vi "Command (read) - IV.vi"(7 "timeout ms (100)":i32=100, 8 "error in (no error)":errorcluster, 9 "Paremeter":string, 10 "IP":string, 11 "connection ID in":refnum<k16>) -> (0 "error out":errorcluster, 2 "Velocity":dbl, 3 "connection ID out":refnum<k16>)   [LabVIEW 2016, in "SMD-7615.lvlib" / "eSCL.lvlib"]
doc: "IV - Immediate Velocity\nRequests present velocity of the motor in rpm. There are two different velocities that can be read back: the\nmotor’s actual velocity and the motor’s target velocity.\nParameter : \n0 = actual velocity request (servo drives and stepper drives with encoder)\n1 = target velocity request"
uses:
  eSCL.lvlib
  DBL Command and Param.ctl
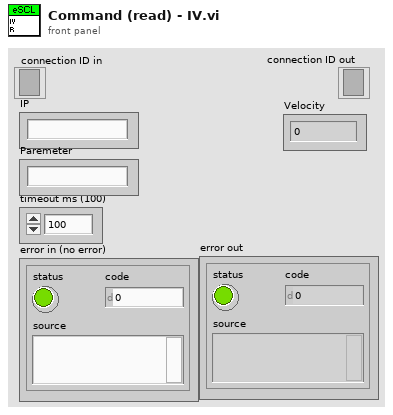
[diagram p1: front panel]
types:
  T1 = typedef "SMD-7615.lvlib/eSCL.lvlib/DBL Command and Param.ctl" = cluster{"Command":string, "DBL Parameler":dbl, "DBL Parameler Default":dbl, "DBL Parameler Coerece Upper":dbl, "DBL Parameler Coerece Lower":dbl}
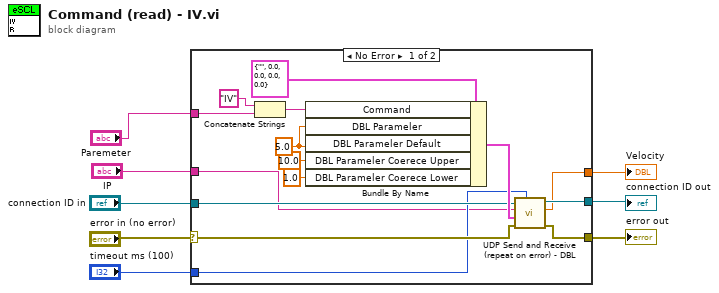
[diagram p0: block diagram]
diagram:
  n1 = case shown="No Error" "error in (no error)" {
    selector: "error in (no error)" -> [w19 w25]
    tunnel: [w18 w24] -> w7
    tunnel: [w17 w25] -> w5
    tunnel: [w16 _] -> w6
    tunnel: "connection ID in" -> [w12 w24]
    tunnel: "timeout ms (100)" -> [w11 _]
    tunnel: "Paremeter" -> [w10 _]
    tunnel: "IP" -> [w9 _]
    frame No Error {
      w15 = 5.0 ("DBL Parameler Default")
      n2 = Concatenate Strings("IV" ("Command"), w10) -> (w13:string)
      n3 = Bundle By Name(cluster=T1 {"Command"="", "DBL Parameler"=0.0, "DBL Parameler Default"=0.0, "DBL Parameler Coerece Upper"=0.0, "DBL Parameler Coerece Lower"=0.0} ("DBL Command & Param"), "Command"=w13, "DBL Parameler"=w15, "DBL Parameler Default"=w15, "DBL Parameler Coerece Upper"=10.0, "DBL Parameler Coerece Lower"=1.0) -> (w20:T1)
      n4 = call "UDP Send and Receive (repeat on error) - DBL.vi"("timeout ms (100)"=w11, "error in (no error)"=w19, "DBL Command & Param"=w20, "IP"=w9, "connection ID in"=w12) -> ("error out"=w17:errorcluster, "DBL Param out"=w16:dbl, "connection ID out"=w18:refnum<k16>)  [unwired: 4 in]
    }
    frame Error {
    }
  }
  "connection ID out" <- w7
  "error out" <- w5
  "Velocity" <- w6
